vi "Get Debug Attribute.vi"(8 "error in (no error)":errorcluster, 11 "SMO":refnum<class "SMO.lvclass">) -> (0 "error out":errorcluster, 2 "Attribute.Debug":refnum<class "Attribute.Debug.lvclass">, 3 "SMO out":refnum<class "SMO.lvclass">)   [LabVIEW 2019, in "Debug.lvlib" / "SMO.Mediator.lvclass"]
uses:
  SMO.Mediator.lvclass
  <vilib>/JKI/JKI SMO/SMO/SMO.lvclass
  Attribute.Debug/Attribute.Debug.lvclass
  C:/Program Files/National Instruments/LabVIEW 2019/vi.lib/JKI/JKI SMO/Support/Attribute/Attribute.lvclass
  <vilib>/JKI/JKI SMO/Support/Attribute/Attribute.lvclass/Attribute.ctl
  <vilib>/Utility/LVClass/Get LV Class Name.vi
  <vilib>/JKI/JKI SMO/Support/Attribute/Attribute.lvclass
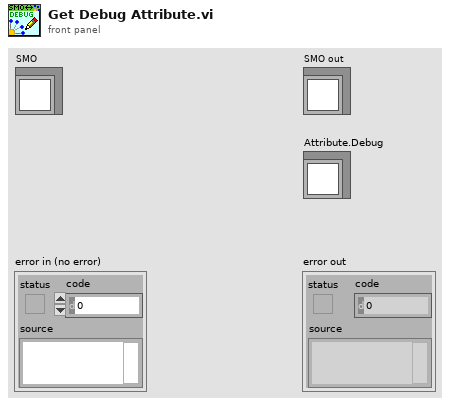
[diagram p1: front panel]
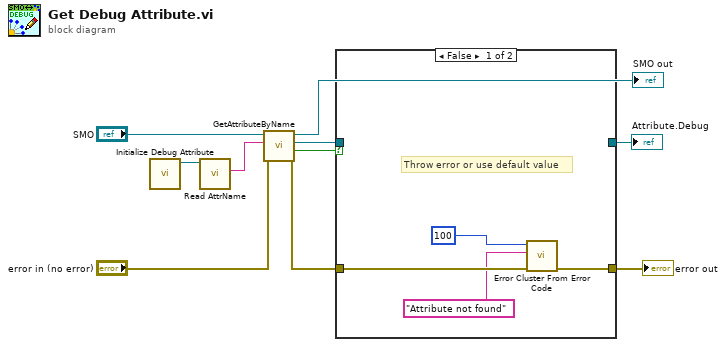
[diagram p0: block diagram]
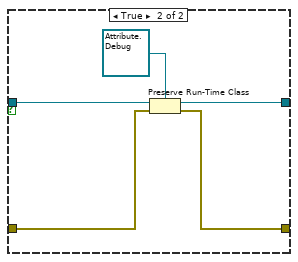
[diagram p2: hidden frame]
diagram:
  n1 = call "Initialize Debug Attribute.vi"() -> ("Attribute.Debug out"=w3:refnum<class "Attribute.Debug.lvclass">)  [unwired: 11 in]
  n2 = call <vilib>:"Read AttrName.vi"("Attribute in"=w3) -> ("Attribute Name"=w2:string)  [unwired: 8 in, 2 out]
  n3 = call <vilib>:"GetAttributeByName.vi"("error in (no error)"="error in (no error)", "AttrName"=w2, "SMO in"="SMO") -> ("error out"=w4:errorcluster, "found"=w7:bool, "Attribute"=w9:refnum<class "Attribute.lvclass">, "SMO out"=→"SMO out":refnum<class "SMO.lvclass">)  [unwired: 5 in]
  n4 = case shown="False" w7 {
    tunnel: w9 -> [_ w19]
    tunnel: [_ w17] -> w8
    tunnel: [w14 w16] -> w5
    tunnel: w4 -> [w13 w15]
    frame False {
      # "Throw error or use default value"
      n5 = call <vilib>:"Error Cluster From Error Code.vi"("error in (no error)"=w13, "error message (\"\")"="Attribute not found" ("error message (\"\")"), "error code (0)"=100) -> ("error out"=w14:errorcluster)  [unwired: 6 in]
    }
    frame True {
      n6 = Preserve Run-Time Class(object in=w19, error in=w15, 2:refnum<class "Attribute.Debug.lvclass"> refnum ("SMO Debug.lvlib:Attribute.Debug.lvclass")) -> (object out=w17:refnum<class "Attribute.Debug.lvclass">, error out=w16:errorcluster)
    }
  }
  "error out" <- w5
  "Attribute.Debug" <- w8
